vi "Evaluate.vi"(0 "object in":refnum<class "ShotTime.lvclass">, 1 "Game":refnum<class "Game.lvclass">, 2 "Point":dbl[](array[numeric]), 3 "Ally?":bool, 5 "error in (no error)":errorcluster) -> (14 "object out":refnum<class "ShotTime.lvclass">, 16 "Evaluation":dbl, 19 "error out":errorcluster)   [LabVIEW 2023, in "ShotTime.lvclass"]
uses:
  ShotTime.lvclass
  Game_class/Game.lvclass
  Game_class/Game.lvclass/Game.ctl
  Field_class/Field.lvclass/Field.ctl
  Team_class/Team.lvclass/Team.ctl
  Referee_class/Referee.lvclass/Referee.ctl
  Object_class/Object.lvclass/Object.ctl
  Game_class/Read Utilities.lvclass.vi
  Game_class/Read FieldRef.vi
  Game_class/Read EnemyRef.vi
  Game_class/Read Referee.vi
  Referee_class/Read enemy_goalie_id.vi
  Team_class/Read RobotRef.vi
  Field_class/Read enemyGoalPosition.vi
  Object_class/Read position(x,y).vi
  Enemy_class/Enemy.lvclass
  C:/Users/ebert/Documents/codes/SSL/repo/SSL_AI/Team_class/Team.lvclass
  Robot_class/Robot.lvclass
  C:/Users/ebert/Documents/codes/SSL/repo/SSL_AI/Object_class/Object.lvclass
  Utilities_class/Utilities.lvclass
  Field_class/Field.lvclass
  Referee_class/Referee.lvclass
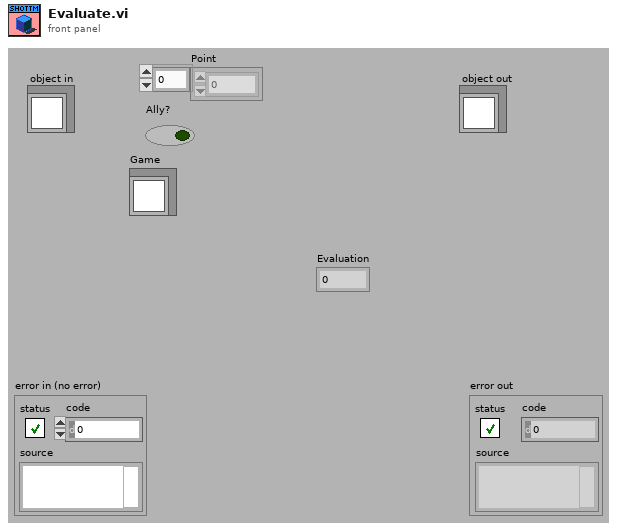
[diagram p1: front panel]
types:
  T1 = typedef "STPParameters.ctl" = cluster{"Skills":T2, "TestSkill":T4, "Events":cluster{"distanceToBallPossession":dbl, "timeForPossessionThreshold":dbl}, "Criteria":cluster{"OpenAngleToGoal":cluster{"minAngle":dbl, "maxAngle":dbl, "minEvaluation":dbl}, "PassDistance":cluster{"maxDistance":dbl, "minDistance":dbl}, "ShotTime":cluster{"shotSpeed":dbl, "keeperSpeed":dbl, "maxShotDistance":dbl, "minEvaluation":dbl}, "OneTouchShot":cluster{"MaxAngle":dbl, "minEvaluation":dbl}}}
  T2 = typedef "Skills.ctl" = cluster{"CirculateBall":T3, "ProtectBall":cluster{"DistanceFromBall":dbl}}
  T3 = typedef "CIrculateSkillParameters.ctl" = cluster{"rotationAngle":dbl, "velocityFactor":dbl, "OrientationFactor":dbl}
  T4 = typedef "TestSkills.ctl" = enum16{"AlignSkill", "PassSkill", "CirculateBall", "OneTouchShotSkill", "KickToSkill_v2", "ShootSkill", "InterceptBall", "GoToSkill_v2"}
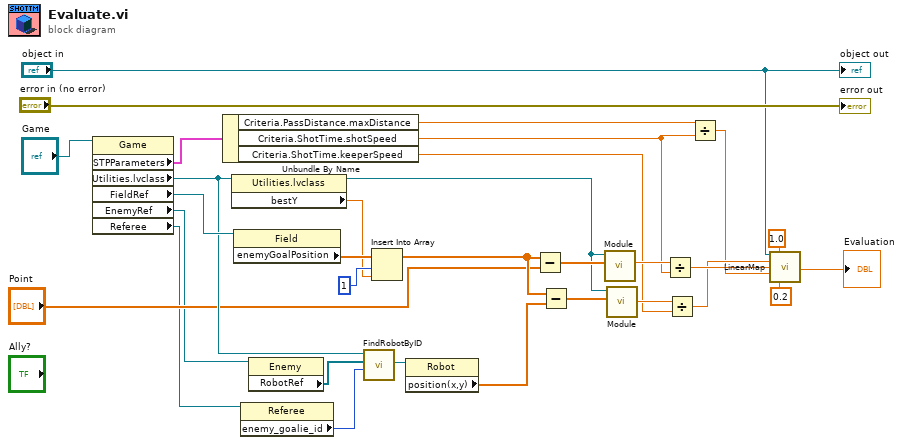
[diagram p0: block diagram]
diagram:
  n1 = property class="Game"(reference="Game") -> ("STPParameters"=w25:T1, "Utilities.lvclass"=w18:refnum<class "Utilities.lvclass">, "FieldRef"=w24:refnum<class "Field.lvclass">, "EnemyRef"=w11:refnum<class "Enemy.lvclass">, "Referee"=w10:refnum<class "Referee.lvclass">)  [unwired: 1 in, 2 out]
  n2 = Unbundle By Name(w25) -> ("Criteria.PassDistance.maxDistance"=w9:dbl, "Criteria.ShotTime.shotSpeed"=w8:dbl, "Criteria.ShotTime.keeperSpeed"=w14:dbl)
  n3 = property class="Utilities.lvclass"(reference=w18) -> (reference out=w17:refnum<class "Utilities.lvclass">, "bestY"=w21:dbl)  [unwired: 1 in, 1 out]
  n4 = property class="Field"(reference=w24) -> ("enemyGoalPosition"=w23:dbl[])  [unwired: 1 in, 2 out]
  n5 = property class="Referee"(reference=w10) -> ("enemy_goalie_id"=w28:i32)  [unwired: 1 in, 2 out]
  n6 = property class="Enemy"(reference=w11) -> ("RobotRef"=w27:refnum<class "Robot.lvclass">[])  [unwired: 1 in, 2 out]
  n7 = call "FindRobotByID.vi"("id"=w28, "RobotRef"=w27, "Utilities in"=w18) -> ("Robot"=w26:refnum<class "Robot.lvclass">)  [unwired: 5 in, 3 out]
  n8 = Insert Into Array(array=w23, index=1, new element=w21) -> (w20:dbl[])
  n9 = property class="Robot"(reference=w26) -> ("position(x,y)"=w19:dbl[])  [unwired: 1 in, 2 out]
  n10 = Subtract(x=w20, y="Point") -> (x-y=w30:dbl[])
  n11 = Subtract(x=w20, y=w19) -> (x-y=w16:dbl[])
  n12 = call "Module.vi"("2D vector"=w30, "Utilities in"=w17) -> ("Modulo"=w29:dbl)  [unwired: 7 in, 2 out]
  n13 = call "Module.vi"("2D vector"=w16, "Utilities in"=w17) -> ("Modulo"=w15:dbl)  [unwired: 7 in, 2 out]
  n14 = Divide(x=w29, y=w8) -> (x/y=w5:dbl)
  n15 = Divide(x=w15, y=w14) -> (x/y=w4:dbl)
  n16 = Divide(x=w9, y=w8) -> (x/y=w3:dbl)
  n17 = call-dynamic "LinearMap.vi"("Criterion in"="object in", "MaxEvalutation"=1.0, "MaxVal"=w4, "Val"=w5, "MinVal"=w3, "MinEvaluation"=0.2) -> ("Evaluation"=→"Evaluation":dbl)  [unwired: 7 in, 2 out]
  "error out" <- "error in (no error)"
  "object out" <- "object in"
